vi "test_libssh2_session_last_errno.vi"() -> ()   [LabVIEW 2017, in "unit_tests.lvlib"]
uses:
  unit_tests.lvlib
  libssh2/libssh2_init_default.vi
  libssh2/libssh2_session_init_ex.vi
  libssh2/libssh2.lvlib
  <vilib>/PNR/Transparent Assertions/Transparent Assertions/Transparent Assertions.lvlib
panel:
  out "error out":errorcluster
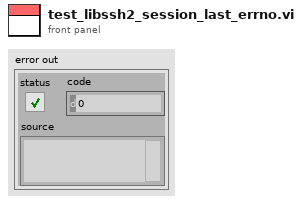
[diagram p1: front panel]
types:
  T1 = typedef "libssh2.lvlib/Session Refnum.ctl" = refnum<k1>
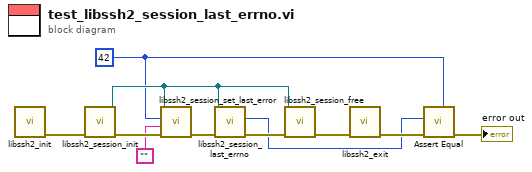
[diagram p0: block diagram]
diagram:
  w3 = 42 ("timeout in ms (0 = indefinite)")
  n1 = call-poly "libssh2_init.vi"() -> ("error out"=w11:errorcluster)  [unwired: 11 in]
  n2 = call "libssh2_session_init.vi"("error in (no error)"=w11) -> ("error out"=w4:errorcluster, "session"=w6:T1)  [unwired: 9 in]
  n3 = call "libssh2_session_set_last_error.vi"("error in (no error)"=w4, "error message"="", "error code"=w3, "session"=w6) -> ("error out"=w9:errorcluster)  [unwired: 7 in]
  n4 = call "libssh2_session_last_errno.vi"("error in (no error)"=w9, "session"=w6) -> ("error out"=w7:errorcluster, "error code"=w5:i32)  [unwired: 8 in]
  n5 = call "libssh2_session_free.vi"("error in (no error)"=w7, "session"=w6) -> ("error out"=w10:errorcluster)  [unwired: 9 in]
  n6 = call "libssh2_exit.vi"("error in (no error)"=w10) -> ("error out"=w8:errorcluster)  [unwired: 10 in]
  n7 = call <vilib>:"Assert Equal.vi"("Expected"=w3, "error in (no error)"=w8, "Actual"=w5) -> ("error out"=→"error out":errorcluster)  [unwired: 8 in]
